vi "gugudan Client.vi"() -> ()   [LabVIEW 2014]
uses:
  <vilib>/Utility/sysdir.llb/System Directory Type.ctl
  <vilib>/FTP/NI_FTP.lvlib
panel:
  out "ip address 3":string=" ip address\r\n   서브넷 마스크 . . . . . . . : 255.255.255.0\r\n   기본 게이트웨이 . . . . . . : 192.168.0.1\r\n\r\n터널 어댑터 isatap.{E2E91750-802C-47E4-94E7-F6C5BD44A78B}:\r\n\r\n   미디어 상태 . . . . . . . . : 미디어 연결 끊김\r\n   연결별 DNS 접미사. . . . : \r\n\r\n터널 어댑터 로컬 영역 연결* 2:\r\n\r\n   연결별 DNS 접미사. . . . : \r\n   IPv6 주소 . . . . . . . . . : 2001:0:682f:9980:3c40:17a9:3f57:fff6\r\n   링크-로컬 IPv6 주소 . . . . : fe80::3c40:17a9:3f57:fff6%12\r\n   기본 게이트웨이 . . . . . . : ::\r\n"
  out "*(타입 *) &x":string
  out "email 2":string
  in  "제한해제":bool
  out "TIME":string="현재날자,시간"
  out "배열":string[][](array[string])
  out "email":string
  out "abs(x)":i32
  out "문자열":string
  out "W":string
  out "D":string
  out "A":string
  out "1":string
  out "2":string
  out "3":string
  out "스페이스바3":string
  # "서비스를 이용해 주셔 감사합니다."
  # "서비스 종료를 위해서는 관리자 암호를 입력 해야 종료가 가능합니다."
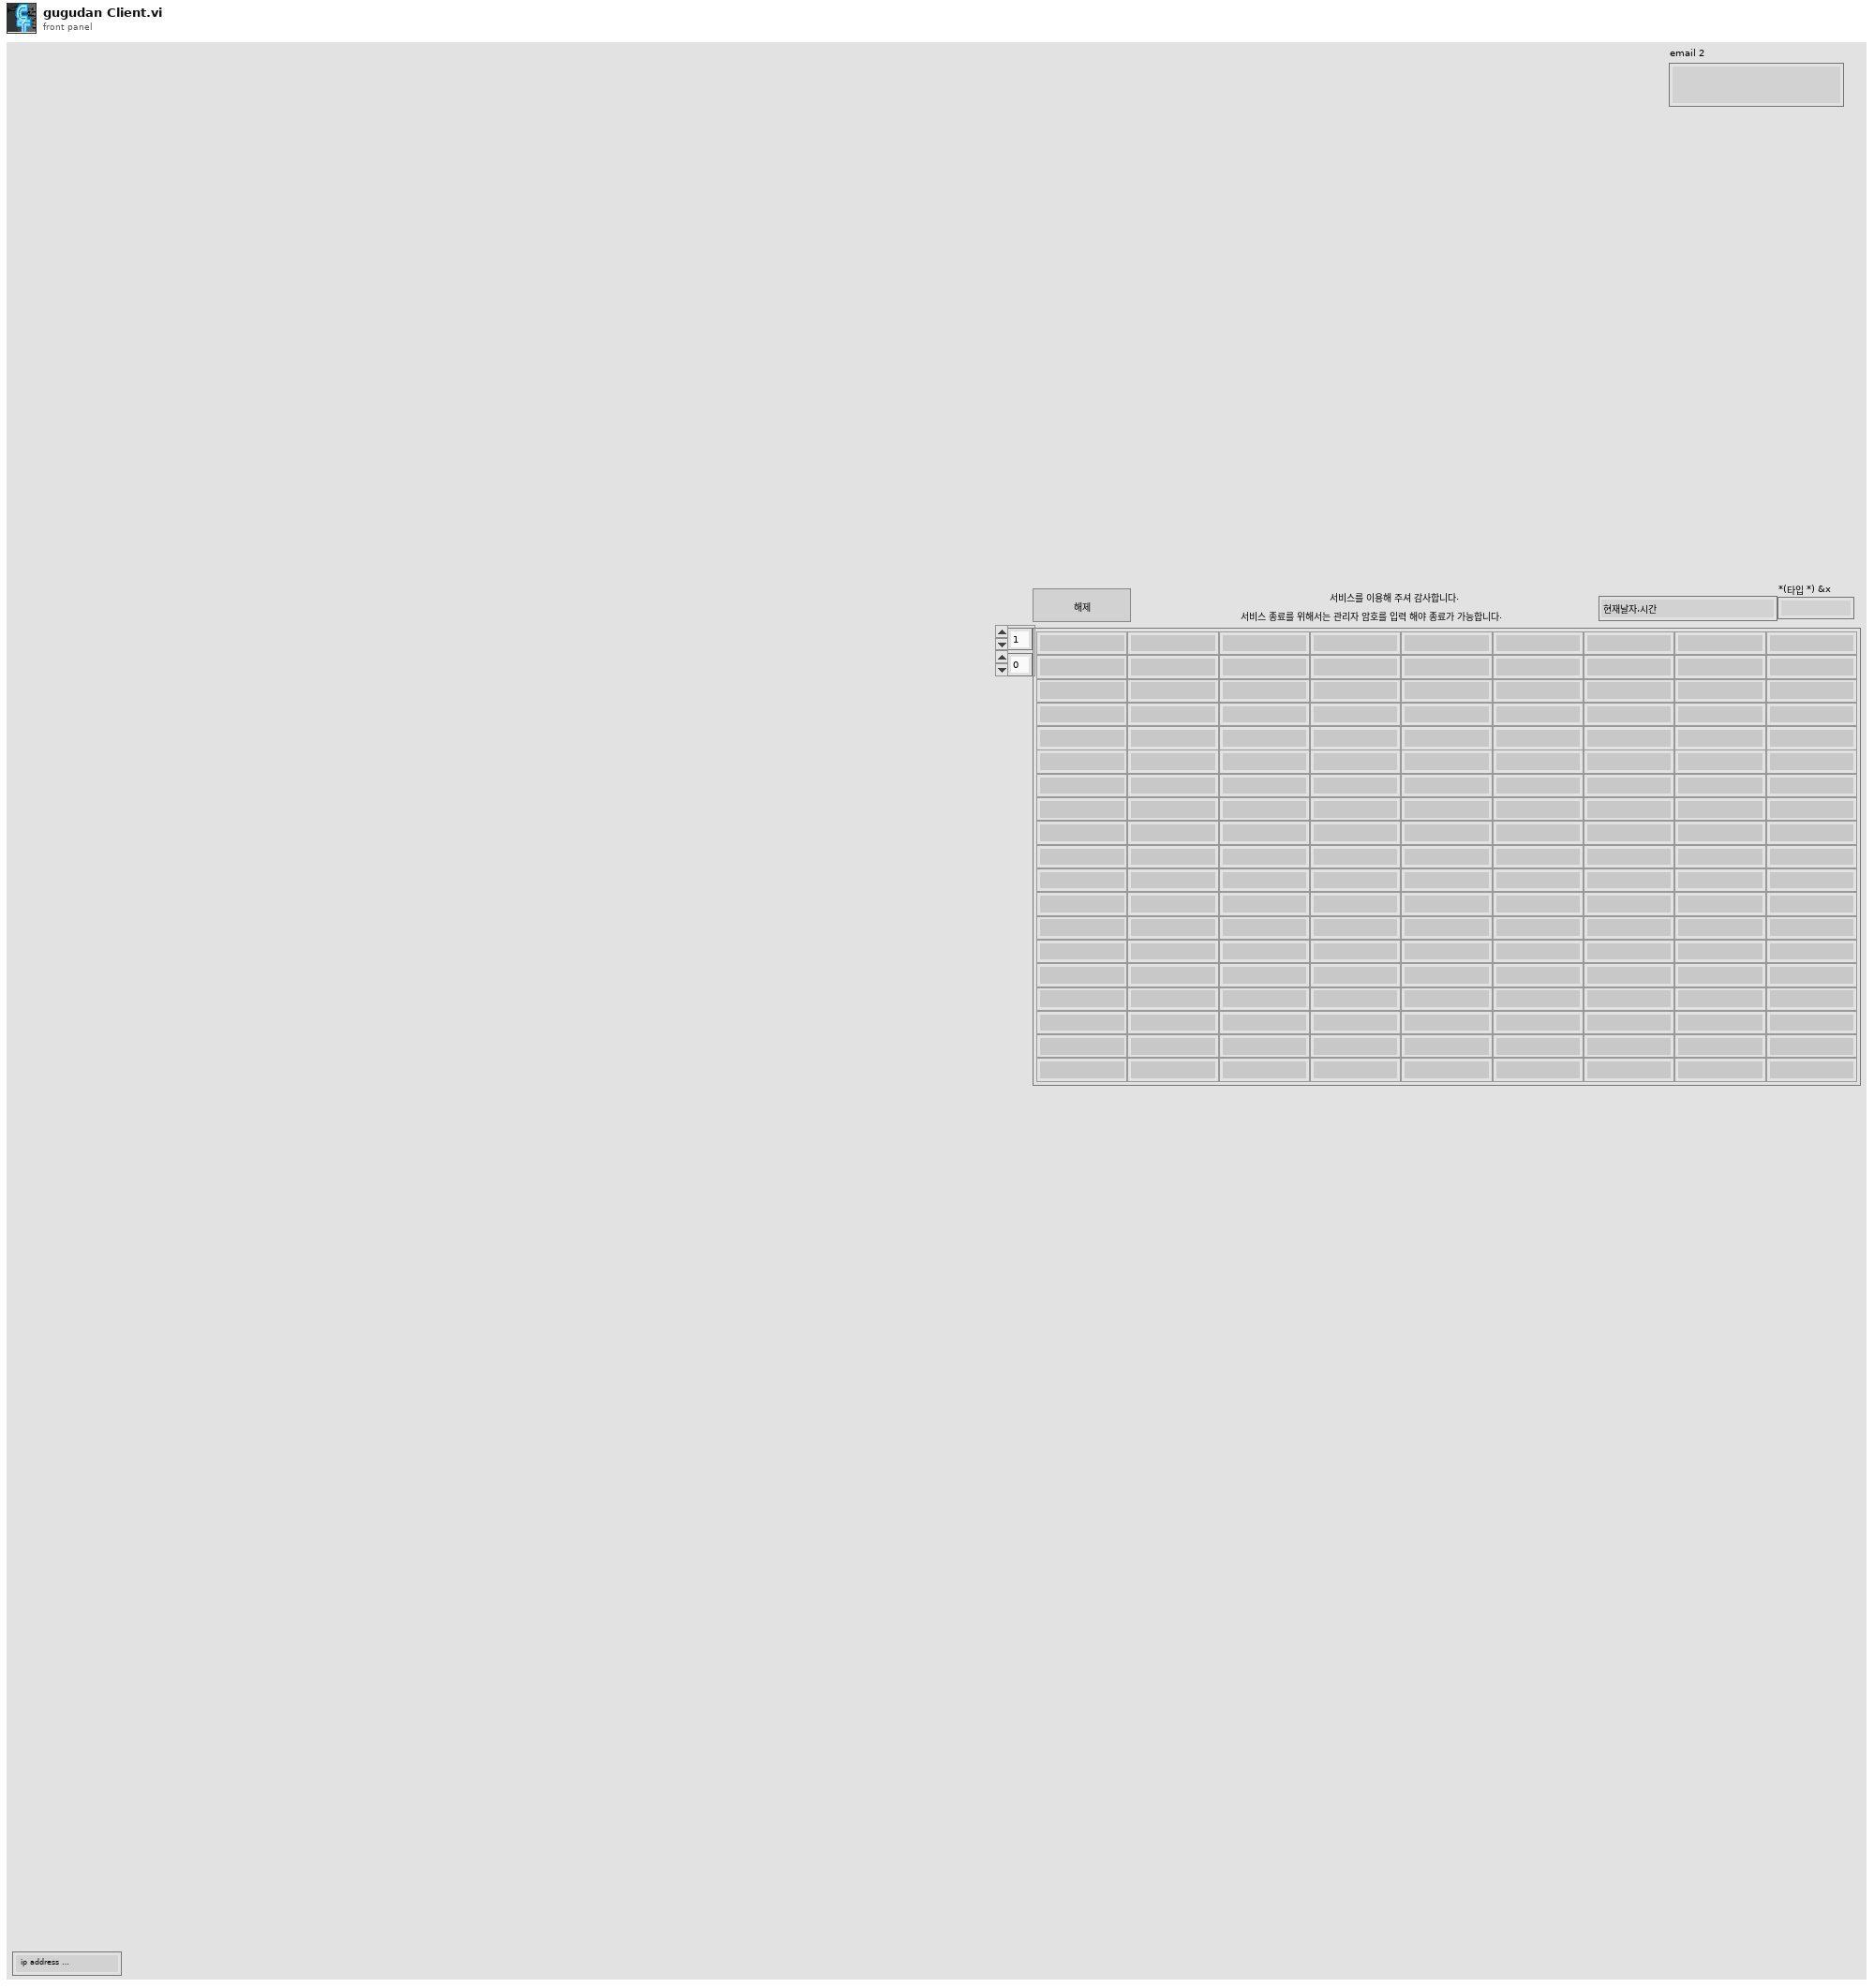
[diagram p1: front panel]
types:
  T1 = enum16{"open", "replace", "create", "open or create", "replace or create", "replace or create with confirmation"}
  T2 = typedef "NI_FTP.lvlib/FTP Session.ctl" = refnum<k5>
  T3 = typedef "System Directory Type.ctl" = i32
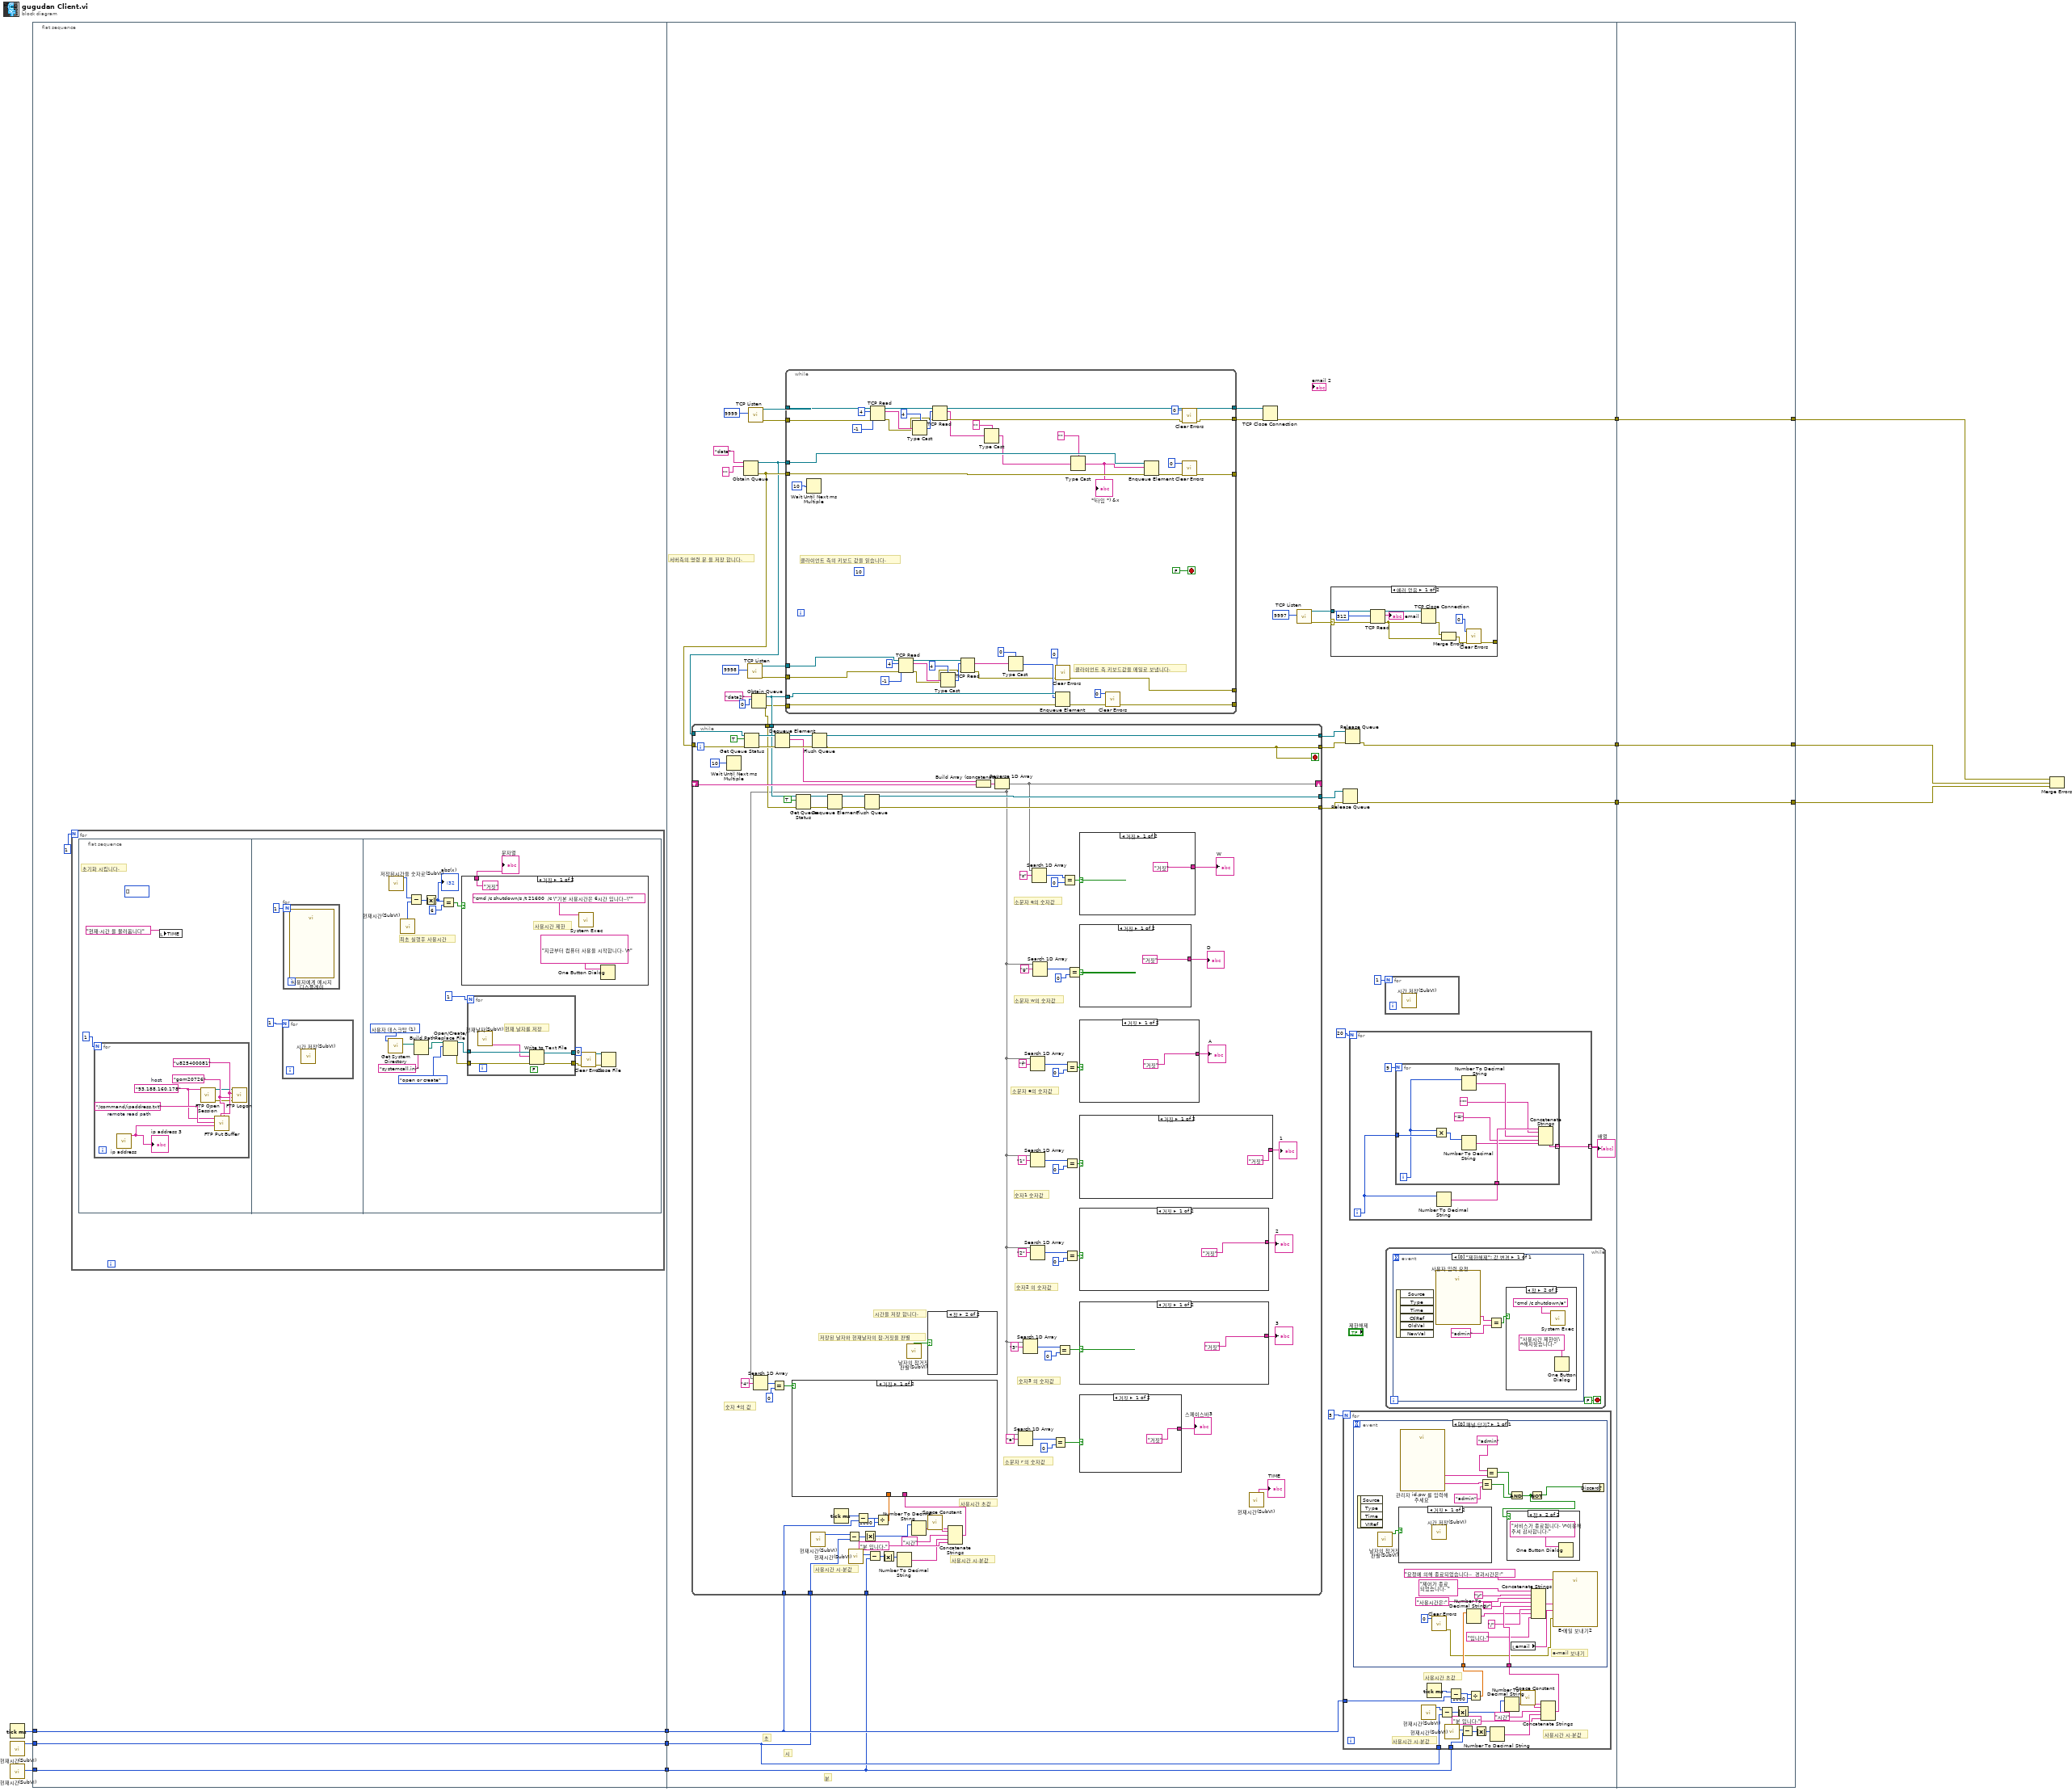
[diagram p0: block diagram]
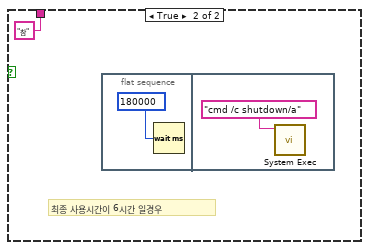
[diagram p2: hidden frame]
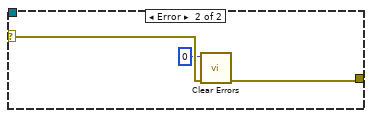
[diagram p4: hidden frame]
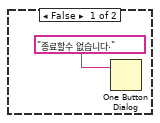
[diagram p6: hidden frame]
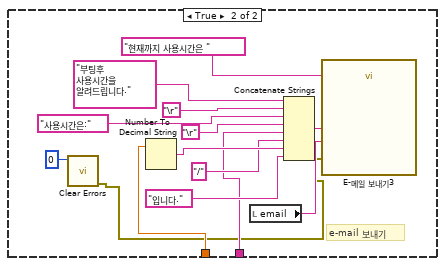
[diagram p7: hidden frame]
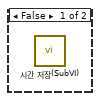
[diagram p8: hidden frame]
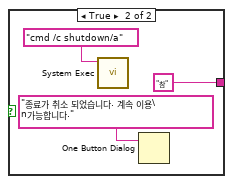
[diagram p9: hidden frame]
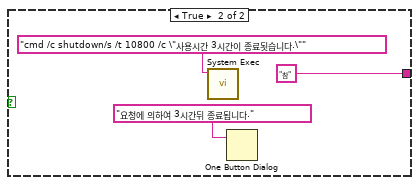
[diagram p10: hidden frame]
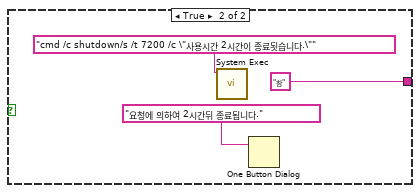
[diagram p11: hidden frame]
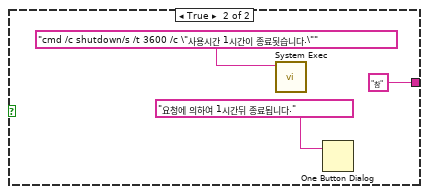
[diagram p12: hidden frame]
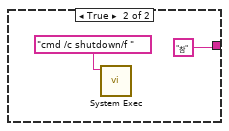
[diagram p13: hidden frame]
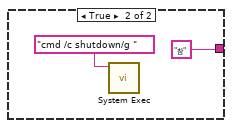
[diagram p14: hidden frame]
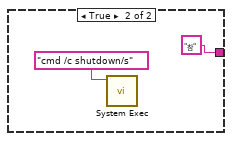
[diagram p15: hidden frame]
diagram:
  n1 = Tick Count (ms)() -> (millisecond timer value=w6:u32)
  n2 = call "현재시간(SubVI).vi"() -> ("시"=w5:i32)  [unwired: 3 in, 8 out]
  n3 = call "현재시간(SubVI).vi"() -> ("분"=w4:i32)  [unwired: 3 in, 8 out]
  n4 = flat-sequence {
    tunnel: [w15] -> w7
    tunnel: w6 -> [w15]
    tunnel: w5 -> [w14]
    tunnel: w4 -> [w13]
    tunnel: [w14] -> w3
    tunnel: [w13] -> w2
    tunnel: [w73] -> w12
    tunnel: [w69] -> w11
    tunnel: [w72] -> w10
    tunnel: w7 -> [w67]
    tunnel: w3 -> [w66]
    tunnel: w2 -> [w65]
    tunnel: w12 -> [w336]
    tunnel: w11 -> [w335]
    tunnel: w10 -> [w334]
    tunnel: [w336] -> w9
    tunnel: [w335] -> w8
    tunnel: [w334] -> w1
    frame #0 {
      n5 = for {
        N: 1 -> [_]
        n6 = flat-sequence {
          frame #0 {
            (unwired) i16[] []
            # "초기화 시킵니다."
            n7 = for {
              N: 1 -> [_]
              w21 = "gom20726"
              w24 = "u825400081"
              w23 = "/command/ipaddress.txt"  # remote read path
              w22 = "93.188.160.178"  # host
              n8 = call "ip address.vi"() -> ("ip address"=w25:string)  [unwired: 11 in]
              "ip address 3" <- w25
              n9 = call <vilib>:"FTP Open Session.vi"("address"=w22) -> ("error out"=w20:errorcluster, "ftp session"=w19:T2)  [unwired: 7 in, 2 out]
              n10 = call <vilib>:"FTP Put Buffer.vi"("password"=w21, "user"=w24, "data"=w25, "remote path"=w23, "host"=w22) -> ()  [unwired: 5 in, 2 out]
              n11 = call <vilib>:"FTP Logon.vi"("error in (no error)"=w20, "password"=w21, "user"=w24, "ftp session"=w19) -> ()  [unwired: 4 in, 4 out]
            }
            n12 = local write "TIME"("현재,시간 을 불러옵니다") -> ()
          }
          frame #1 {
            n13 = for {
              N: 1 -> [_]
              n14 = call "시간 저장(SubVI).vi"() -> ()  [unwired: 12 in]
            }
            n15 = for {
              N: 1 -> [_]
              n16 = call "사용자에게 메시지 디스플레이"() -> ()  [unwired: 10 in, 2 out]
            }
          }
          frame #2 {
            w30 = T3 1 items=["사용자 홈"=0, "사용자 데스크탑"=1, "사용자 문서"=2, "사용자 어플리케이션 데이터"=3, "사용자 환경"=4, "사용자 임시"=5, "퍼블릭 문서"=6, "퍼블릭 어플리케이션 데이터"=7, "퍼블릭 환경"=8, "퍼블릭 캐시"=13, "시스템 코어 라이브러리"=9, "시스템 설치된 라이브러리"=10, "어플리케이션 파일"=11, "부팅 볼륨 루트"=12] ("system directory type")
            # "최초 실행후 사용시간"
            n17 = call <vilib>:"Get System Directory.vi"("system directory type"=w30) -> ("system directory"=w35:path)  [unwired: 10 in]
            n18 = call "저장된시간을 숫자로(SubVI).vi"() -> ("저장된 문자를 숫자로"=w40:i32)  [unwired: 11 in]
            n19 = call "현재시간(SubVI).vi"() -> ("시"=w41:i32)  [unwired: 3 in, 8 out]
            n20 = Subtract(x=w40, y=w41) -> (x-y=w42:i32)
            n21 = Build Path(base path=w35, name or relative path="systemcall.ini" ("이름 또는 상대 경로")) -> (appended path=w33:path)
            n22 = Absolute Value(x=w42) -> (abs(x)=w44:i32)
            "abs(x)" <- w44
            n23 = Equal?(x=w44, y=6) -> (x = y?=w46:bool)
            n24 = Open/Create/Replace File(file path (use dialog)=w33, operation (0:open)=T1."open or create" ("동작(0:open)")) -> (refnum out=w31:refnum<file>, error out=w32:errorcluster)  [unwired: 4 in, 1 out]
            n25 = case shown="거짓" w46 {
              tunnel: ["거짓" "참"] -> w43
              frame False {
                # "사용시간 제한"
                n26 = call <vilib>:"System Exec.vi"("command line"="cmd /c shutdown/s /t 21600  /c \"기본 사용시간은 6시간 입니다..\"" ("standard input")) -> ()  [unwired: 7 in, 4 out]
                n27 = One Button Dialog(message="지금부터 컴퓨터 사용을 시작합니다. \n" ("메시지")) -> ()  [unwired: 1 in, 1 out]
              }
              frame True {
                # "최종 사용시간이 6시간 일경우"
                n28 = flat-sequence {
                  frame #0 {
                    n29 = Wait (ms)(milliseconds to wait=u32 180000 ("대기 시간(ms)")) -> ()  [unwired: 1 out]
                  }
                  frame #1 {
                    n30 = call <vilib>:"System Exec.vi"("command line"="cmd /c shutdown/a" ("standard input")) -> ()  [unwired: 7 in, 4 out]
                  }
                }
              }
            }
            "문자열" <- w43
            n31 = for {
              N: 1 -> [_]
              tunnel: w32 -> [w51]
              tunnel: [w50] -> w37
              tunnel: [w49] -> w36
              tunnel: w31 -> [w48]
              (unwired) FALSE
              # "현재 날자를 저장"
              n32 = call "현재날자(SubVI).vi"() -> ("월,일 을 문자열로"=w47:string)  [unwired: 5 in, 6 out]
              n33 = Write to Text File(file (use dialog)=w48, text=w47, error in=w51) -> (refnum out=w49:refnum<file>, error out=w50:errorcluster)  [unwired: 1 in, 1 out]
            }
            n34 = call <vilib>:"Clear Errors.vi"("error in (no error)"=w37, "specific error code to clear (0: all)"=0) -> ("error out"=w38:errorcluster)  [unwired: 4 in, 1 out]
            n35 = Close File(refnum=w36, error in=w38) -> ()  [unwired: 2 out]
          }
        }
      }
    }
    frame #1 {
      # "서버측의 명령 문 을 저장 합니다."
      # "초"
      # "분"
      # "시"
      n36 = Obtain Queue(name (unnamed)="data" ("이름(이름없음)"), element data type="") -> (queue out=w83:refnum<queue>, error out=w84:errorcluster)  [unwired: 3 in, 1 out]
      n37 = call <vilib>:"TCP Listen.vi"("port"=u16 9998) -> ("error out"=w80:errorcluster, "connection ID"=w81:refnum<k5>)  [unwired: 6 in, 3 out]
      n38 = call <vilib>:"TCP Listen.vi"("port"=u16 9999) -> ("error out"=w70:errorcluster, "connection ID"=w88:refnum<k5>)  [unwired: 6 in, 3 out]
      n39 = Obtain Queue(name (unnamed)="data2" ("이름(이름없음)"), element data type=i16 0) -> (queue out=w75:refnum<queue>, error out=w74:errorcluster)  [unwired: 3 in, 1 out]
      n40 = while {
        shift-right: [w176] -> _
        shift-left: _ -> [w220]
        tunnel: [w213] -> w86
        tunnel: [w212] -> w85
        tunnel: w83 -> [w219]
        tunnel: w84 -> [w218]
        tunnel: [w203] -> w77
        tunnel: [w202] -> w76
        tunnel: w75 -> [w201]
        tunnel: w74 -> [w200]
        tunnel: w67 -> [w181]
        tunnel: w66 -> [w180]
        tunnel: w65 -> [w179]
        stop <- w212 stop-if-true
        # "숫자 4의 값"
        # "저장된 날자와 현재날자의 참,거짓을 판별"
        # "시간을 저장 합니다."
        # "사용시간 시,분값"
        # "사용시간 시,분값"
        # "사용시간 초값"
        # "소문자 r 의 숫자값"
        # "숫자3 의 숫자값"
        # "소문자 q의 숫자값"
        # "소문자 w의 숫자값"
        # "소문자 e의 숫자값"
        # "숫자1 숫자값"
        # "숫자2 의 숫자값"
        n41 = Wait Until Next ms Multiple(millisecond multiple=u32 10) -> ()  [unwired: 1 out]
        n42 = Get Queue Status(queue=w219, return elements? (F)=TRUE ("원소 반환? (거짓)"), error in (no error)=w218) -> (queue out=w217:refnum<queue>, error out=w216:errorcluster)  [unwired: 6 out]
        n43 = Dequeue Element(queue=w217, error in (no error)=w216) -> (queue out=w214:refnum<queue>, element=w211:string, error out=w215:errorcluster)  [unwired: 1 in, 1 out]
        n44 = Get Queue Status(queue=w201, return elements? (F)=TRUE ("원소 반환? (거짓)"), error in (no error)=w200) -> (queue out=w207:refnum<queue>, error out=w206:errorcluster)  [unwired: 6 out]
        n45 = call "현재시간(SubVI).vi"() -> ("시"=w183:i32)  [unwired: 3 in, 8 out]
        n46 = Flush Queue(queue=w214, error in (no error)=w215) -> (queue out=w213:refnum<queue>, error out=w212:errorcluster)  [unwired: 1 out]
        n47 = Dequeue Element(queue=w207, error in (no error)=w206) -> (queue out=w204:refnum<queue>, error out=w205:errorcluster)  [unwired: 1 in, 2 out]
        n48 = Tick Count (ms)() -> (millisecond timer value=w182:u32)
        n49 = Subtract(x=w183, y=w180) -> (x-y=w185:i32)
        n50 = call "현재시간(SubVI).vi"() -> ("분"=w184:i32)  [unwired: 3 in, 8 out]
        n51 = Subtract(x=w182, y=w181) -> (x-y=w194:u32)
        n52 = Absolute Value(x=w185) -> (abs(x)=w187:i32)
        n53 = Flush Queue(queue=w204, error in (no error)=w205) -> (queue out=w202:refnum<queue>, error out=w203:errorcluster)  [unwired: 1 out]
        n54 = Subtract(x=w184, y=w179) -> (x-y=w186:i32)
        n55 = Divide(x=w194, y=u32 1000) -> (x/y=w178:dbl)
        n56 = Absolute Value(x=w186) -> (abs(x)=w188:i32)
        n57 = Number To Decimal String(number=w188) -> (decimal integer string=w190:string)  [unwired: 1 in]
        n58 = call "날자의 참거짓 판별(SubVI).vi"() -> ("불리언"=w199:bool)  [unwired: 9 in, 2 out]
        n59 = Number To Decimal String(number=w187) -> (decimal integer string=w192:string)  [unwired: 1 in]
        n60 = call <vilib>:"Space Constant.vi"() -> ("String"=w193:string)
        n61 = case shown="참" w199 {
          frame False {
            n62 = call "시간 저장(SubVI).vi"() -> ()  [unwired: 12 in]
          }
          frame True {
          }
        }
        n63 = Concatenate Strings(w192, w193, "시간", w190, "분 입니다.") -> (w177:string)
        n64 = Build Array (concatenate)(w211, w220) -> (w209:string[])
        n65 = Reverse 1D Array(array=w209) -> (reversed array=w176:string[])
        n66 = Search 1D Array(1D array=w176, element="4" ("원소")) -> (index of element=w198:i32)  [unwired: 1 in]
        n67 = Equal?(x=w198, y=0) -> (x = y?=w196:bool)
        n68 = case shown="거짓" w196 {
          tunnel: w178 -> [_ w254]
          tunnel: w177 -> [_ w253]
          frame False {
          }
          frame True {
            # "e-mail 보내기"
            n69 = call <vilib>:"Clear Errors.vi"("specific error code to clear (0: all)"=0) -> ("error out"=w250:errorcluster)  [unwired: 5 in, 1 out]
            n70 = Number To Decimal String(number=w254) -> (decimal integer string=w262:string)  [unwired: 1 in]
            n71 = local read "email"() -> (w252:string)
            n72 = Concatenate Strings("부팅후 사용시간을 알려드립니다." ("문자열"), "\r", "사용시간은:", "\r", w253, "/", w262, "입니다.") -> (w259:string)
            n73 = call "E-메일 보내기3"("error in"=w250, "Message"=w259, "Subject"="현재까지 사용시간은 ", "Recipients"=w252) -> ()  [unwired: 7 in, 1 out]
          }
        }
        n74 = Search 1D Array(1D array=w176, element="a" ("원소")) -> (index of element=w224:i32)  [unwired: 1 in]
        n75 = Search 1D Array(1D array=w176, element="3" ("원소")) -> (index of element=w229:i32)  [unwired: 1 in]
        n76 = Search 1D Array(1D array=w176, element="f" ("원소")) -> (index of element=w238:i32)  [unwired: 1 in]
        n77 = Search 1D Array(1D array=w176, element="1" ("원소")) -> (index of element=w237:i32)  [unwired: 1 in]
        n78 = Search 1D Array(1D array=w176, element="2" ("원소")) -> (index of element=w230:i32)  [unwired: 1 in]
        n79 = Search 1D Array(1D array=w176, element="s" ("원소")) -> (index of element=w248:i32)  [unwired: 1 in]
        n80 = Search 1D Array(1D array=w176, element="g" ("원소")) -> (index of element=w246:i32)  [unwired: 1 in]
        n81 = Equal?(x=w224, y=0) -> (x = y?=w226:bool)
        n82 = Equal?(x=w229, y=0) -> (x = y?=w227:bool)
        n83 = Equal?(x=w248, y=0) -> (x = y?=w245:bool)
        n84 = Equal?(x=w238, y=0) -> (x = y?=w240:bool)
        n85 = Equal?(x=w237, y=0) -> (x = y?=w235:bool)
        n86 = Equal?(x=w230, y=0) -> (x = y?=w232:bool)
        n87 = Equal?(x=w246, y=0) -> (x = y?=w243:bool)
        n88 = case shown="거짓" w245 {
          tunnel: ["거짓" "참"] -> w249
          frame False {
          }
          frame True {
            n89 = call <vilib>:"System Exec.vi"("command line"="cmd /c shutdown/s" ("standard input")) -> ()  [unwired: 7 in, 4 out]
          }
        }
        "W" <- w249
        n90 = case shown="거짓" w243 {
          tunnel: ["거짓" "참"] -> w244
          frame False {
          }
          frame True {
            n91 = call <vilib>:"System Exec.vi"("command line"="cmd /c shutdown/g " ("standard input")) -> ()  [unwired: 7 in, 4 out]
          }
        }
        "D" <- w244
        n92 = case shown="거짓" w240 {
          tunnel: ["거짓" "참"] -> w239
          frame False {
          }
          frame True {
            n93 = call <vilib>:"System Exec.vi"("command line"="cmd /c shutdown/f " ("standard input")) -> ()  [unwired: 7 in, 4 out]
          }
        }
        "A" <- w239
        n94 = case shown="거짓" w235 {
          tunnel: ["거짓" "참"] -> w236
          frame False {
          }
          frame True {
            n95 = call <vilib>:"System Exec.vi"("command line"="cmd /c shutdown/s /t 3600 /c \"사용시간 1시간이 종료됫습니다.\"" ("standard input")) -> ()  [unwired: 7 in, 4 out]
            n96 = One Button Dialog(message="요청에 의하여 1시간뒤 종료됩니다." ("메시지")) -> ()  [unwired: 1 in, 1 out]
          }
        }
        "1" <- w236
        n97 = case shown="거짓" w232 {
          tunnel: ["거짓" "참"] -> w231
          frame False {
          }
          frame True {
            n98 = call <vilib>:"System Exec.vi"("command line"="cmd /c shutdown/s /t 7200 /c \"사용시간 2시간이 종료됫습니다.\"" ("standard input")) -> ()  [unwired: 7 in, 4 out]
            n99 = One Button Dialog(message="요청에 의하여 2시간뒤 종료됩니다." ("메시지")) -> ()  [unwired: 1 in, 1 out]
          }
        }
        "2" <- w231
        n100 = case shown="거짓" w227 {
          tunnel: ["거짓" "참"] -> w210
          frame False {
          }
          frame True {
            n101 = call <vilib>:"System Exec.vi"("command line"="cmd /c shutdown/s /t 10800 /c \"사용시간 3시간이 종료됫습니다.\"" ("standard input")) -> ()  [unwired: 7 in, 4 out]
            n102 = One Button Dialog(message="요청에 의하여 3시간뒤 종료됩니다." ("메시지")) -> ()  [unwired: 1 in, 1 out]
          }
        }
        "3" <- w210
        n103 = case shown="거짓" w226 {
          tunnel: ["거짓" "참"] -> w223
          frame False {
          }
          frame True {
            n104 = call <vilib>:"System Exec.vi"("command line"="cmd /c shutdown/a" ("standard input")) -> ()  [unwired: 7 in, 4 out]
            n105 = One Button Dialog(message="종료가 취소 되었습니다. 계속 이용\n가능합니다." ("메시지")) -> ()  [unwired: 1 in, 1 out]
          }
        }
        "스페이스바3" <- w223
        n106 = call "현재시간(SubVI).vi"() -> ("날짜/시간 문자열"=→"TIME":string)  [unwired: 3 in, 8 out]
      }
      n107 = while {
        tunnel: w88 -> [w294]
        tunnel: [w333] -> w89
        tunnel: w83 -> [w326]
        tunnel: w84 -> [w325]
        tunnel: w81 -> [w295]
        tunnel: w80 -> [w316]
        tunnel: w75 -> [w311]
        tunnel: w74 -> [w312]
        tunnel: [w307] -> w71
        tunnel: w70 -> [w308]
        tunnel: [w304] -> _
        tunnel: [w300] -> _
        tunnel: [w297] -> _
        stop <- FALSE stop-if-true
        (unwired) 10
        # "클라이언트 측 키보드값을 메일로 보냅니다."
        # "클라이언트 측의 키보드 값을 읽습니다."
        n108 = Wait Until Next ms Multiple(millisecond multiple=u32 10) -> ()  [unwired: 1 out]
        n109 = TCP Read(connection ID=w294, bytes to read=4, error in (no error)=w308, 9:-1 ("타임아웃 ms (25000)")) -> (connection ID out=w329:refnum<k5>, data out=w331:string, error out=w309:errorcluster)  [unwired: 1 in]
        n110 = TCP Read(connection ID=w295, bytes to read=4, error in (no error)=w316, 9:-1 ("타임아웃 ms (25000)")) -> (connection ID out=w319:refnum<k5>, data out=w317:string, error out=w315:errorcluster)  [unwired: 1 in]
        n111 = Type Cast(type=4 ("bytes to read"), x=w331) -> (*(type *) &x=w324:i32)
        n112 = TCP Read(connection ID=w329, bytes to read=w324, error in (no error)=w309) -> (connection ID out=w333:refnum<k5>, data out=w291:string, error out=w306:errorcluster)  [unwired: 2 in]
        n113 = Type Cast(type=4 ("bytes to read"), x=w317) -> (*(type *) &x=w322:i32)
        n114 = TCP Read(connection ID=w319, bytes to read=w322, error in (no error)=w315) -> (data out=w314:string, error out=w298:errorcluster)  [unwired: 2 in, 1 out]
        n115 = Type Cast(type="", x=w291) -> (*(type *) &x=w290:string)
        n116 = Type Cast(type=i16 0, x=w314) -> (*(type *) &x=w310:i16)
        n117 = Enqueue Element(queue=w311, element=w310, error in (no error)=w312) -> (error out=w301:errorcluster)  [unwired: 1 in, 2 out]
        n118 = call <vilib>:"Clear Errors.vi"("error in (no error)"=w298, "specific error code to clear (0: all)"=0) -> ("error out"=w297:errorcluster)  [unwired: 4 in, 1 out]
        n119 = Type Cast(type="", x=w290) -> (*(type *) &x=w292:string)
        "*(타입 *) &x" <- w292
        n120 = call <vilib>:"Clear Errors.vi"("error in (no error)"=w301, "specific error code to clear (0: all)"=0) -> ("error out"=w300:errorcluster)  [unwired: 4 in, 1 out]
        n121 = Enqueue Element(queue=w326, element=w292, error in (no error)=w325) -> (error out=w305:errorcluster)  [unwired: 1 in, 2 out]
        n122 = call <vilib>:"Clear Errors.vi"("error in (no error)"=w306, "specific error code to clear (0: all)"=0) -> ("error out"=w307:errorcluster)  [unwired: 4 in, 1 out]
        n123 = call <vilib>:"Clear Errors.vi"("error in (no error)"=w305, "specific error code to clear (0: all)"=0) -> ("error out"=w304:errorcluster)  [unwired: 4 in, 1 out]
      }
      n124 = TCP Close Connection(connection ID=w89, error in (no error)=w71) -> (error out=w72:errorcluster)  [unwired: 1 in, 1 out]
      n125 = call <vilib>:"TCP Listen.vi"("port"=u16 9997) -> ("error out"=w62:errorcluster, "connection ID"=w63:refnum<k5>)  [unwired: 6 in, 3 out]
      n126 = case shown="에러 없음" w62 {
        selector: w62 -> [w115 w121]
        tunnel: [w112 w122] -> _
        tunnel: w63 -> [w119 _]
        frame No Error {
          n127 = TCP Read(connection ID=w119, bytes to read=512, error in (no error)=w115) -> (connection ID out=w114:refnum<k5>, data out=→"email":string, error out=w113:errorcluster)  [unwired: 2 out]
          n128 = TCP Close Connection(connection ID=w114, error in (no error)=w113) -> (error out=w116:errorcluster)  [unwired: 2 out]
          n129 = Merge Errors(w116, w113) -> (w111:errorcluster)
          n130 = call <vilib>:"Clear Errors.vi"("error in (no error)"=w111, "specific error code to clear (0: all)"=0) -> ("error out"=w112:errorcluster)  [unwired: 4 in, 1 out]
        }
        frame Error {
          n131 = call <vilib>:"Clear Errors.vi"("error in (no error)"=w121, "specific error code to clear (0: all)"=0) -> ("error out"=w122:errorcluster)  [unwired: 4 in, 1 out]
        }
      }
      n132 = Release Queue(queue=w76, error in (no error)=w77) -> (error out=w69:errorcluster)  [unwired: 1 in, 2 out]
      n133 = for {
        N: 5 -> [_]
        tunnel: w67 -> [w140]
        tunnel: w66 -> [w138]
        tunnel: w65 -> [w136]
        # "사용시간 시,분값"
        # "사용시간 시,분값"
        # "사용시간 초값"
        n134 = call "현재시간(SubVI).vi"() -> ("시"=w139:i32)  [unwired: 3 in, 8 out]
        n135 = Tick Count (ms)() -> (millisecond timer value=w141:u32)
        n136 = Subtract(x=w139, y=w138) -> (x-y=w135:i32)
        n137 = call "현재시간(SubVI).vi"() -> ("분"=w137:i32)  [unwired: 3 in, 8 out]
        n138 = Subtract(x=w141, y=w140) -> (x-y=w126:u32)
        n139 = Absolute Value(x=w135) -> (abs(x)=w133:i32)
        n140 = Subtract(x=w137, y=w136) -> (x-y=w134:i32)
        n141 = Divide(x=w126, y=u32 1000) -> (x/y=w124:dbl)
        n142 = Absolute Value(x=w134) -> (abs(x)=w132:i32)
        n143 = Number To Decimal String(number=w132) -> (decimal integer string=w130:string)  [unwired: 1 in]
        n144 = Number To Decimal String(number=w133) -> (decimal integer string=w128:string)  [unwired: 1 in]
        n145 = call <vilib>:"Space Constant.vi"() -> ("String"=w127:string)
        n146 = Concatenate Strings(w128, w127, "시간", w130, "분 입니다.") -> (w123:string)
        n147 = event shown="[0] 패널 닫기?" {
          selector: _ -> [_]
          dyn-events: _ -> [_]
          timeout: _ -> [_]
          tunnel: w124 -> [w156]
          tunnel: w123 -> [w149]
          event Panel Close? {
            # "e-mail 보내기"
            n148 = event-data() -> ()  [unwired: 1 in, 4 out]
            n149 = call "날자의 참거짓 판별(SubVI).vi"() -> ("불리언"=w145:bool)  [unwired: 9 in, 2 out]
            n150 = case shown="거짓" w145 {
              frame False {
                n151 = call "시간 저장(SubVI).vi"() -> ()  [unwired: 12 in]
              }
              frame True {
              }
            }
            n152 = call "관리자 id.pw 를 입력해 주세요"() -> ("PW"=w164:string, "ID"=w161:string)  [unwired: 16 in, 2 out]
            n153 = call <vilib>:"Clear Errors.vi"("specific error code to clear (0: all)"=0) -> ("error out"=w143:errorcluster)  [unwired: 5 in, 1 out]
            n154 = Number To Decimal String(number=w156) -> (decimal integer string=w147:string)  [unwired: 1 in]
            n155 = Equal?(x=w164, y="admin") -> (x = y?=w160:bool)
            n156 = Equal?(x="admin", y=w161) -> (x = y?=w159:bool)
            n157 = And(x=w159, y=w160) -> (x .and. y?=w157:bool)
            n158 = case shown="참" w157 {
              frame False {
                n159 = One Button Dialog(message="종료할수 없습니다." ("메시지")) -> ()  [unwired: 1 in, 1 out]
              }
              frame True {
                n160 = One Button Dialog(message="서비스가 종료됩니다. \n이용해 주셔 감사합니다." ("메시지")) -> ()  [unwired: 1 in, 1 out]
              }
            }
            n161 = local read "email"() -> (w144:string)
            n162 = Not(x=w157) -> (.not. x?=w158:bool)
            n163 = Concatenate Strings("제어가 종료 되었습니다. " ("문자열"), "\r", "사용시간은:", "\r", w149, "/", w147, "입니다.") -> (w151:string)
            n164 = call "E-메일 보내기2"("error in"=w143, "Message"=w151, "Subject"="요청에 의해 종료되었습니다,.  경과시간은:", "Recipients"=w144) -> ()  [unwired: 7 in, 1 out]
            n165 = event-data("Discard?"=w158) -> ()  [unwired: 1 in, 1 out]
          }
        }
      }
      n166 = Release Queue(queue=w86, error in (no error)=w85) -> (error out=w73:errorcluster)  [unwired: 1 in, 2 out]
      n167 = for {
        N: 20 -> [_]
        tunnel: [w97] -> w60 mode=indexing
        i -> [w99]
        n168 = Number To Decimal String(number=w99) -> (decimal integer string=w98:string)  [unwired: 1 in]
        n169 = for {
          N: 9 -> [_]
          tunnel: w99 -> [w109]
          tunnel: w98 -> [w107]
          tunnel: [w102] -> w97 mode=indexing
          i -> [w101]
          n170 = Multiply(x=w101, y=w109) -> (x*y=w108:i32)
          n171 = Number To Decimal String(number=w101) -> (decimal integer string=w106:string)  [unwired: 1 in]
          n172 = Number To Decimal String(number=w108) -> (decimal integer string=w103:string)  [unwired: 1 in]
          n173 = Concatenate Strings(w107, "*", w106, "=", w103) -> (w102:string)
        }
      }
      "배열" <- w60
      n174 = for {
        N: 1 -> [_]
        n175 = call "시간 저장(SubVI).vi"() -> ()  [unwired: 12 in]
      }
      n176 = while {
        stop <- FALSE stop-if-true
        n177 = event shown="[0] \"제한해제\": 값 변경" {
          selector: _ -> [_]
          dyn-events: _ -> [_]
          timeout: _ -> [_]
          event "제한해제": Value Change {
            n178 = event-data() -> ()  [unwired: 1 in, 6 out]
            n179 = call "사용자 입력 요청"() -> ("종료 취소"=w93:string)  [unwired: 17 in, 2 out]
            n180 = Equal?(x=w93, y="admin") -> (x = y?=w92:bool)
            n181 = case shown="참" w92 {
              frame False {
              }
              frame True {
                n182 = call <vilib>:"System Exec.vi"("command line"="cmd /c shutdown/a" ("standard input")) -> ()  [unwired: 7 in, 4 out]
                n183 = One Button Dialog(message="사용시간 제한이\n해지됫습니다." ("메시지")) -> ()  [unwired: 1 in, 1 out]
              }
            }
          }
        }
      }
    }
    frame #2 {
    }
  }
  n184 = Merge Errors(w1, w9, w8) -> ()  [unwired: 1 out]
